vi "Read Config File.vi"(8 "error in (no error)":errorcluster, 11 "Air Cooler Application in":refnum<class "Air Cooler Application.lvclass">) -> (0 "error out":errorcluster, 3 "Air Cooler Application out":refnum<class "Air Cooler Application.lvclass">)   [LabVIEW 2018, in "Air Cooler Application.lvlib" / "Air Cooler Application.lvclass"]
doc: "This VI reads the configuration file associated with this application and populates the application object with the information therein. For any keys that are not found in the configuration file, the default value is specified by setting the default values of the private data control."
uses:
  Air Cooler Application.lvclass
  Air Cooler Application.lvclass/Air Cooler Application.ctl
  <vilib>/Utility/config.llb/NI_LVConfig.lvlib
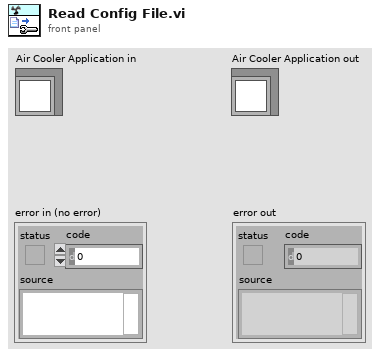
[diagram p1: front panel]
types:
  T1 = typedef "NI_LVConfig.lvlib/Config Data RefNum.ctl" = refnum<k1>
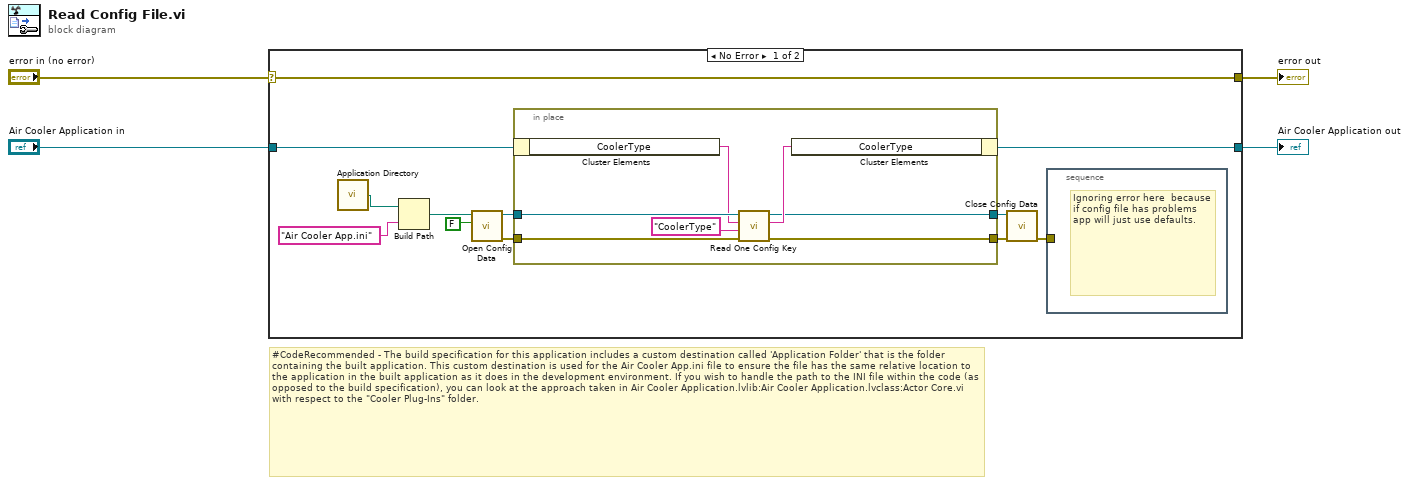
[diagram p0: block diagram]
diagram:
  # "#CodeRecommended - The build specification for this application includes a custom destination called 'Application Folder' that is the folder containing the built application. This custom destination is used for the Air Cooler App.ini file to ensure the file has the same relative location to the application in the built application as it does in the development environment. If you wish to handle the path to the INI file within the code (as opposed to the build specification), you can look at the approach taken in Air Cooler Application.lvlib:Air Cooler Application.lvclass:Actor Core.vi with respect to the \"Cooler Plug-Ins\" folder."
  n1 = case shown="No Error" "error in (no error)" {
    selector: "error in (no error)" -> [w10 w25]
    tunnel: [w10 w25] -> w3
    tunnel: [w8 w24] -> w1
    tunnel: "Air Cooler Application in" -> [w9 w24]
    frame No Error {
      n2 = call <vilib>:"Application Directory.vi"() -> ("Application Directory"=w16:path)
      n3 = Build Path(base path=w16, name or relative path="Air Cooler App.ini") -> (appended path=w5:path)
      n4 = call <vilib>:"Open Config Data.vi"("create file if necessary (T)"=FALSE, "configuration file path"=w5) -> ("error out"=w13:errorcluster, "refnum"=w12:T1)  [unwired: 7 in, 1 out]
      n5 = in-place {
        in-place-border: w13 -> [w23]
        in-place-border: w12 -> [w22]
        in-place-border: [w17] -> w7
        in-place-border: [w18] -> w6
        n6 = in-place-cluster #1(w9) -> ("CoolerType"=w19:string)
        n7 = call "Read One Config Key.vi"("error in (no error)"=w23, "key"="CoolerType", "default value"=w19, "Refnum in"=w22) -> ("error out"=w18:errorcluster, "value"=w20:string, "Refnum out"=w17:T1)  [unwired: 5 in]
        n8 = in-place-cluster #1("CoolerType"=w20) -> (w8:refnum<class "Air Cooler Application.lvclass">)
      }
      n9 = call <vilib>:"Close Config Data.vi"("error in (no error)"=w6, "refnum"=w7) -> ("error out"=w11:errorcluster)  [unwired: 8 in, 1 out]
      n10 = stacked-sequence {
        tunnel: w11 -> [_]
        frame #0 {
          # "Ignoring error here  because if config file has problems app will just use defaults."
        }
      }
    }
    frame Error {
    }
  }
  "error out" <- w3
  "Air Cooler Application out" <- w1
